vi "Free Running Avs47b with temperature display.vi"() -> ()   [LabVIEW 2012]
doc: "Application example"
panel:
  out "VISA RESOURCE":refnum<visa-resource-name>
  out "CALIBRATION FILE [CH]":string[](array[string])
  out "R PAST CALIBR RANGE":bool
  out "TEMPERATURE UNIT":string
  out "TEMPERATURE":dbl
  in  "stop":bool
  out "RESISTANCE":sgl format="%^_6e"
  in  "REMOTE":u8(ring)=1 items=["NO", "YES"]
  in  "DIGITAL REFERENCE":u16 max=19999 step=1
  in  "DISPLAY":u8(ring) items=["R", "DR", "ADJ REF", "REFERENCE", "EXC VOLT", "530A HEAT V", "530A HEAT I", "530A SET PT"]
  in  "EXCITATION":u8(ring)=7 items=["NO EXCITATION", "3 uV", "10uV", "30uV", "100uV", "300uV", "1mV", "3mV"]
  in  "RANGE":u8(ring)=3 items=["NO RANGE", "2 Ohms", "20 Ohms", "200 Ohms", "2 kOhms", "20 kOhms", "200 kOhms", "2 MOhms"]
  in  "CHANNEL":u8(ring) items=["CH0", "CH1", "CH2", "CH3", "CH4", "CH5", "CH6", "CH7"]
  in  "INPUT":u8(ring)=2 items=["ZERO", "MEAS", "CAL"]
  out "ADC OVERRANGE":bool
  # "Free Running Avs47b with temperature display.vi"
  # "RV-Elektroniikka Oy\nPicowatt"
  # "Etc...."
  # "This  example shows, how a continuously running VI can be used for producing both resistance and temperature readouts.  This VI reads the AVS47B configuration file for setting initial values.  These settings can be edited as long as the VI is running. Pressing STOP saves the last configuration and sets the bridge in local mode.\n\nTemperature display requires two  additional files:\n1)  avs47b_rt_file_info.cnf, which contains information about  the format of the R/T calibration \n     (or   conversion) files\n2)  a calibration (conversion) file for each sensor that one wants to be  be displayed also in terms of temperature\n\nRefer to the manual and \"Edit RT Information File.vi\" for how to create these files. This VI package\ncontains also a conversion file for a non-cryogenic  PT-100 sensor. It is a simple text file and can be\nopened with a text editor like Notepad, Textpad etc. If a wordprocessor is used, the file must be\nsaved in plain text format without any formatting characters."
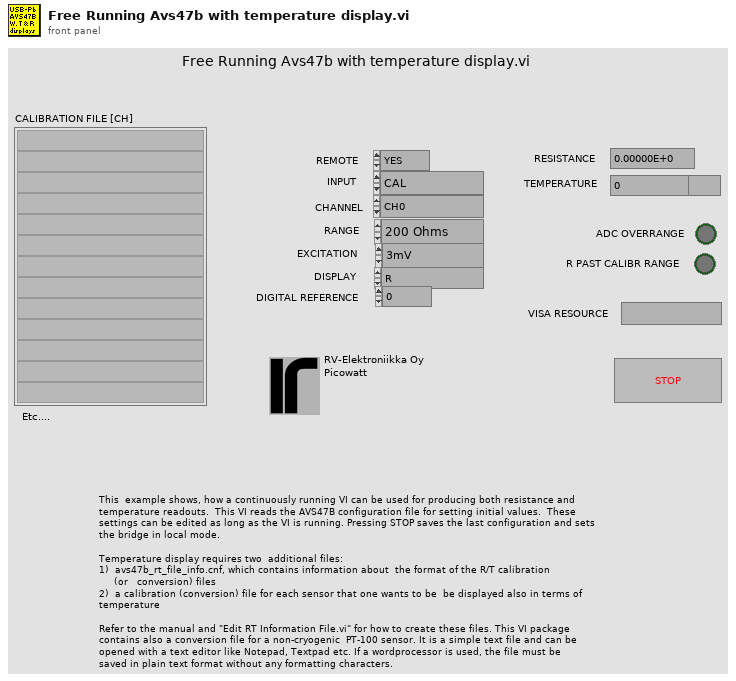
[diagram p1: front panel]
types:
  T1 = enum16{"NONE", "READ", "READ AND EDIT", "DEFAULTS"}
  T2 = cluster{"VISA RESOURCE":refnum<visa-resource-name>, "PICOBUS ADDRESS":u8, "DISABLE AL":u8, "REMOTE":u8, "INPUT":u8, "CHANNEL":u8, "RANGE":u8, "EXCITATION":u8, "DISPLAY":u8, "DIGITAL REFERENCE":u16, "SET POINT":dbl, "PROP GAIN":u8, "INTG":u8, "DERIV":u8, "POWER BIAS":u8, "POWER RANGE":u8, "INFO STRING":string, "HEATER RESISTANCE":dbl, "INTERVAL":u8, " SENSOR dR/dT":u8}
  T3 = cluster{"NUMBER OF POINTS":i32, "SIGN OF dT/dR":enum16{"POSITIVE", "NEGATIVE"}, "R/T FORMAT ":enum16{"R", "LOG(R)"}, "TEMPERATURE SCALE":enum16{"KELVINS", "CELSIUS"}, "FILE OK":i32}[]
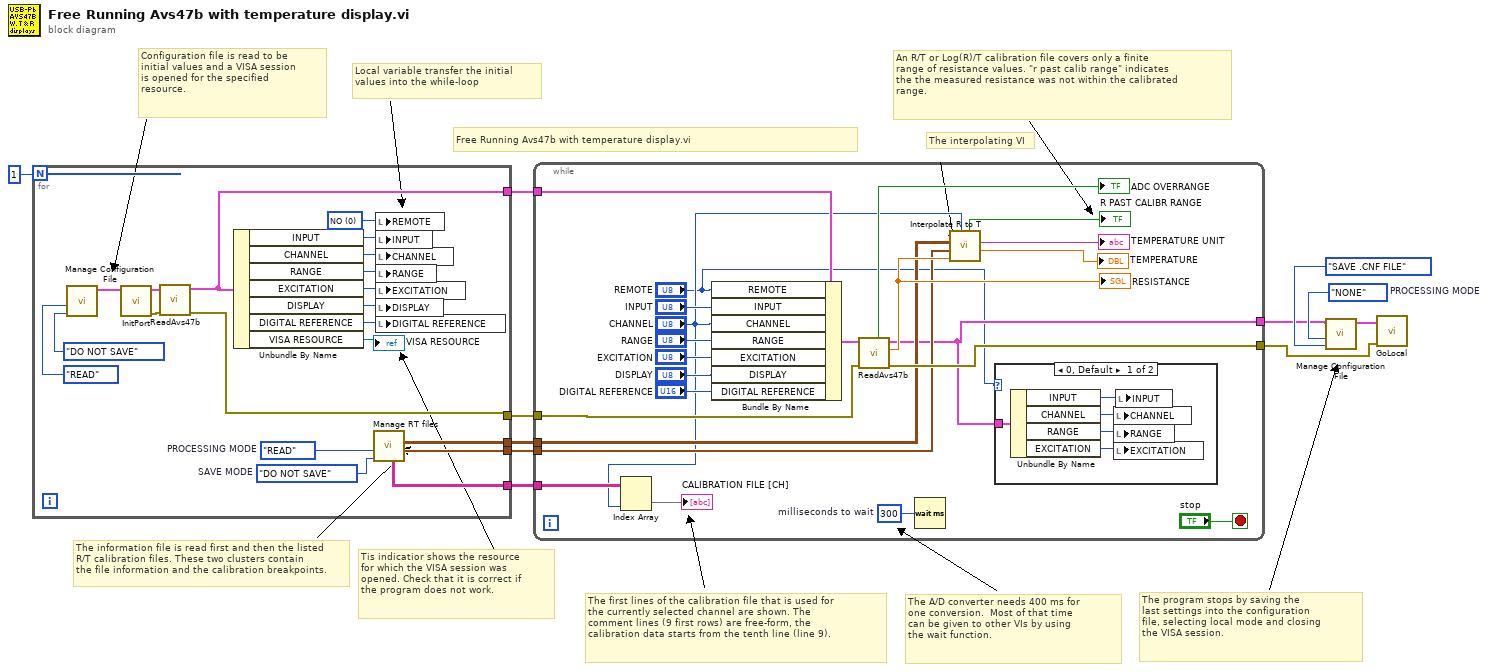
[diagram p0: block diagram]
diagram:
  w5 = enum16{"NONE", "READ", "CREATE"}."NONE"  # PROCESSING MODE
  # "The interpolating VI"
  # "The information file is read first and then the listed\nR/T calibration files. These two clusters contain\nthe file information and the calibration breakpoints."
  # "The program stops by saving the\nlast settings into the configuration\nfile, selecting local mode and closing \nthe VISA session."
  # "The A/D converter needs 400 ms for\none conversion.  Most of that time\ncan be given to other VIs by using \nthe wait function."
  # "An R/T or Log(R)/T calibration file covers only a finite\nrange of resistance values. \"r past calib range\" indicates\nthe the measured resistance was not within the calibrated\nrange."
  # "The first lines of the calibration file that is used for \nthe currently selected channel are shown. The\ncomment lines (9 first rows) are free-form, the\ncalibration data starts from the tenth line (line 9)."
  # "Tis indicatior shows the resource\nfor which the VISA session was \nopened. Check that it is correct if\nthe program does not work."
  # "Local variable transfer the initial\nvalues into the while-loop"
  # "Configuration file is read to be\ninitial values and a VISA session\nis opened for the specified \nresource."
  # "Free Running Avs47b with temperature display.vi"
  n1 = for {
    N: 1 -> [_]
    tunnel: [w21] -> w10
    tunnel: [w20] -> w9
    tunnel: [w25] -> w8
    tunnel: [w24] -> w7
    tunnel: [w23] -> w6
    w12 = enum16{"DO NOT SAVE", "SAVE .CNF FILE"}."DO NOT SAVE"  # SAVE MODE
    w13 = T1."READ"  # PROCESSING MODE
    w19 = u8 0 items=["NO", "YES"] ("REMOTE")
    n2 = call "Manage Configuration File.vi"("SAVE MODE"=enum16{"DO NOT SAVE", "SAVE .CNF FILE"}."DO NOT SAVE", "PROCESSING MODE"=enum16{"NONE", "READ", "CREATE"}."READ") -> ("CONFIGURATION CLUSTER OUT"=w18:T2)  [unwired: 9 in]
    n3 = call "InitPort.vi"("CONFIGURATION CLUSTER"=w18) -> ("LV ERROR OUT"=w15:errorcluster, "UNMODIFIED CONFIGURATION CLUSTER"=w16:T2)  [unwired: 6 in, 1 out]
    n4 = call "ReadAvs47b.vi"("LV ERROR IN"=w15, "CONFIGURATION CLUSTER"=w16) -> ("LV ERROR OUT"=w21:errorcluster, "MODIFIED CONFIGURATION CLUSTER"=w20:T2)  [unwired: 4 in, 4 out]
    n5 = Unbundle By Name(w20) -> ("INPUT"=w31:u8, "CHANNEL"=w30:u8, "RANGE"=w29:u8, "EXCITATION"=w28:u8, "DISPLAY"=w27:u8, "DIGITAL REFERENCE"=w26:u16, "VISA RESOURCE"=→"VISA RESOURCE":refnum<visa-resource-name>)
    n6 = call "Manage RT files.vi"("SAVE MODE"=w12, "PROCESSING MODE"=w13) -> ("FILE INFO"=w24:T3, "R/T BREAKPOINTS"=w25:cluster{dbl, dbl}[][], "COMMENT AREA (9 FIRST ROWS)"=w23:string[][])  [unwired: 5 in, 2 out]
    n7 = local write "REMOTE"(w19) -> ()
    n8 = local write "INPUT"(w31) -> ()
    n9 = local write "CHANNEL"(w30) -> ()
    n10 = local write "RANGE"(w29) -> ()
    n11 = local write "EXCITATION"(w28) -> ()
    n12 = local write "DISPLAY"(w27) -> ()
    n13 = local write "DIGITAL REFERENCE"(w26) -> ()
  }
  n14 = while {
    tunnel: w10 -> [w54]
    tunnel: [w51] -> w1
    tunnel: [w33] -> w3
    tunnel: w9 -> [w45]
    tunnel: w8 -> [w41]
    tunnel: w7 -> [w40]
    tunnel: w6 -> [w36]
    stop <- "stop" stop-if-true
    w53 = u32 300  # milliseconds to wait
    n15 = Index Array(array=w36, index (col)="CHANNEL") -> (element=→"CALIBRATION FILE [CH]":string[])  [unwired: 1 in]
    n16 = Bundle By Name(cluster=w45, "REMOTE"="REMOTE", "INPUT"="INPUT", "CHANNEL"="CHANNEL", "RANGE"="RANGE", "EXCITATION"="EXCITATION", "DISPLAY"="DISPLAY", "DIGITAL REFERENCE"="DIGITAL REFERENCE") -> (w52:T2)
    n17 = call "ReadAvs47b.vi"("LV ERROR IN"=w54, "CONFIGURATION CLUSTER"=w52) -> ("LV ERROR OUT"=w51:errorcluster, "RESISTANCE (OHMS)"=w42:sgl, "MODIFIED CONFIGURATION CLUSTER"=w33:T2, "ADC OVERRANGE"=→"ADC OVERRANGE":bool)  [unwired: 4 in, 2 out]
    "RESISTANCE" <- w42
    n18 = Wait (ms)(milliseconds to wait=w53) -> ()  [unwired: 1 out]
    n19 = call "Interpolate R to T.vi"("CHANNEL"="CHANNEL", "RESISTANCE (OHMS)"=w42, "FILE INFO"=w40, "R/T POINTS"=w41) -> ("TEMPERATURE"=→"TEMPERATURE":dbl, "TEMPERATURE UNIT"=→"TEMPERATURE UNIT":string, "R PAST CALIBRATION RANGE"=→"R PAST CALIBR RANGE":bool)  [unwired: 4 in, 1 out]
    n20 = case shown="0, Default" "REMOTE" {
      tunnel: w33 -> [w59 _]
      frame 0, Default {
        n21 = Unbundle By Name(w59) -> ("INPUT"=w58:u8, "CHANNEL"=w57:u8, "RANGE"=w56:u8, "EXCITATION"=w55:u8)
        n22 = local write "CHANNEL"(w57) -> ()
        n23 = local write "RANGE"(w56) -> ()
        n24 = local write "EXCITATION"(w55) -> ()
        n25 = local write "INPUT"(w58) -> ()
      }
      frame 1 {
      }
    }
  }
  n26 = call "Manage Configuration File.vi"("SAVE MODE"=enum16{"DO NOT SAVE", "SAVE .CNF FILE"}."SAVE .CNF FILE", "PROCESSING MODE"=w5, "CONFIGURATION CLUSTER"=w3) -> ("CONFIGURATION CLUSTER OUT"=w2:T2)  [unwired: 8 in]
  n27 = call "GoLocal.vi"("LV ERROR IN"=w1, "CONFIGURATION CLUSTER"=w2) -> ()  [unwired: 9 in, 1 out]
